vi "Read Unfiltered Log Content.vi"(8 "error in (no error)":errorcluster, 11 "Debug Log In":refnum<class "Debug Log.lvclass">) -> (0 "error out":errorcluster, 2 "Data Log":refnum<class "Debug Data.lvclass">[](array[class]), 3 "Debug Log Out":refnum<class "Debug Log.lvclass">)   [LabVIEW 2020, in "Debug Log.lvclass"]
uses:
  Debug Log.lvclass
  Debug Data/Debug Data.lvclass
  Debug Log.lvclass/Debug Log.ctl
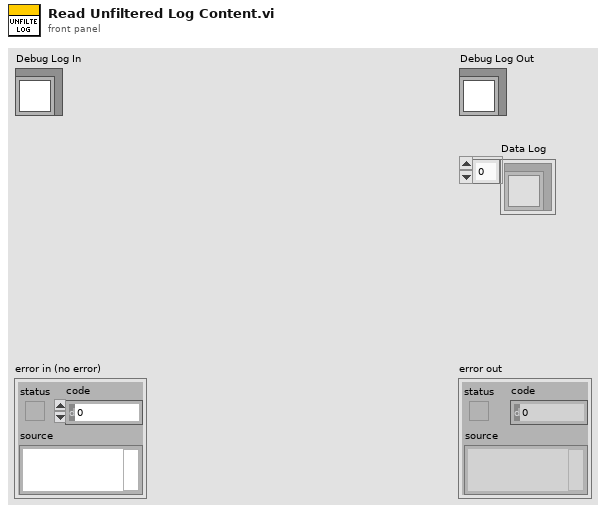
[diagram p1: front panel]
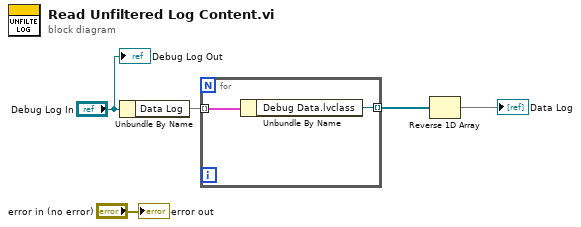
[diagram p0: block diagram]
diagram:
  n1 = Unbundle By Name("Debug Log In") -> ("Data Log"=w2:map{u32, refnum<class "Debug Data.lvclass">})
  n2 = for {
    tunnel: w2 -> [w7] mode=indexing
    tunnel: [w6] -> w3 mode=indexing
    n3 = Unbundle By Name(w7) -> ("Debug Data.lvclass"=w6:refnum<class "Debug Data.lvclass">)
  }
  n4 = Reverse 1D Array(array=w3) -> (reversed array=→"Data Log":refnum<class "Debug Data.lvclass">[])
  "error out" <- "error in (no error)"
  "Debug Log Out" <- "Debug Log In"
